vi "Unknown Signal State Machine.vi"() -> ()   [LabVIEW 2011]
doc: "Use this template to build a standard state machine design pattern. Each state executes code and determines which state to transition to. Contrast this design pattern with the User Interface Event Handler pattern, in which code executes in response to user actions. Contrast this design pattern also with the Queued Message Handler pattern, in which each message handling code can queue zero or more new messages."
uses:
  DAQstates.ctl
  <vilib>/DAQmx/read.llb/DAQmx Read (Analog 1D Wfm NChan NSamp).vi
  <vilib>/DAQmx/create/channels.llb/DAQmx Create Channel (AI-Voltage-Basic).vi
  <vilib>/DAQmx/configure/timing.llb/DAQmx Timing (Sample Clock).vi
  <vilib>/DAQmx/miscellaneous.llb/DAQmx Fill In Error Info.vi
  <vilib>/Waveform/WDTFileIO.llb/Export Waveforms To Spreadsheet File (1D).vi
panel:
  out "Waveform Graph":waveform(dbl)[](graph)
  out "Current State":T1
  in  "Stop":bool
  in  "Save Data":bool
  in  "Take Data":bool
  in  "Channel 2":tag
  in  "samples per channel":i32=1000
  in  "Rate(Hz)":dbl=1000.0 format="%0.2f"
  in  "Channel 1":tag
  out "Error Messages":errorcluster
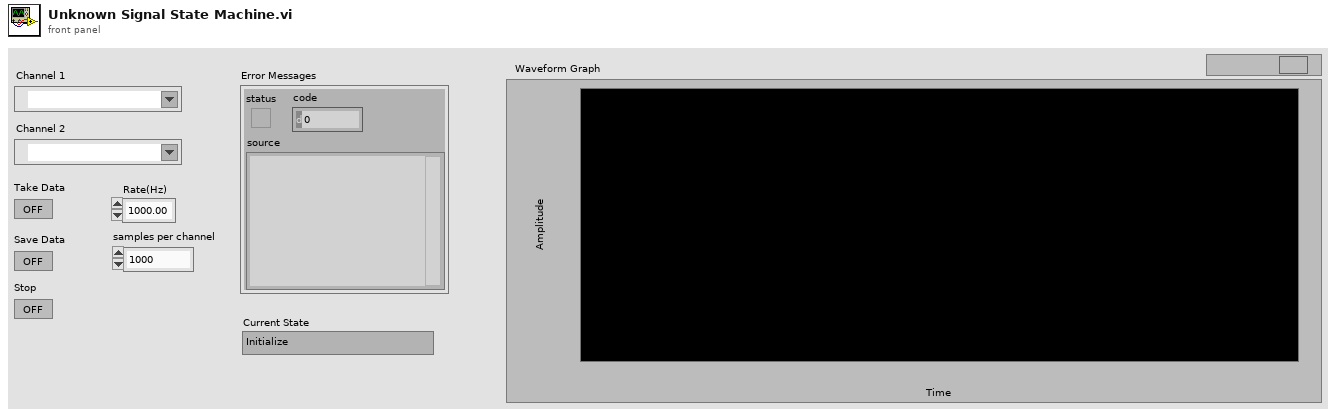
[diagram p1: front panel]
types:
  T1 = typedef "DAQstates.ctl" = enum16{"Initialize", "Wait", "Stop", "Take Data", "Save Data", ""}
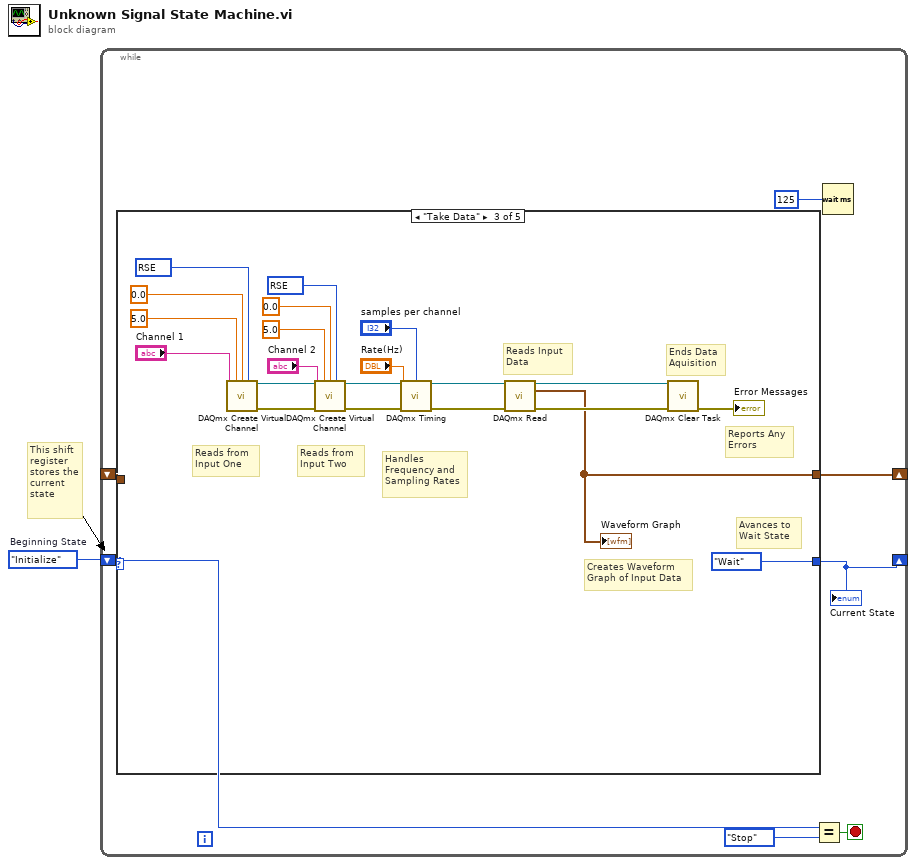
[diagram p0: block diagram]
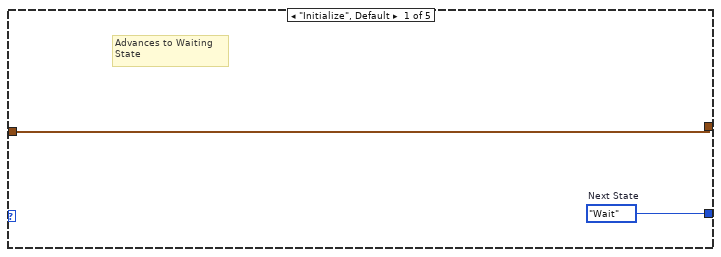
[diagram p2: hidden frame]
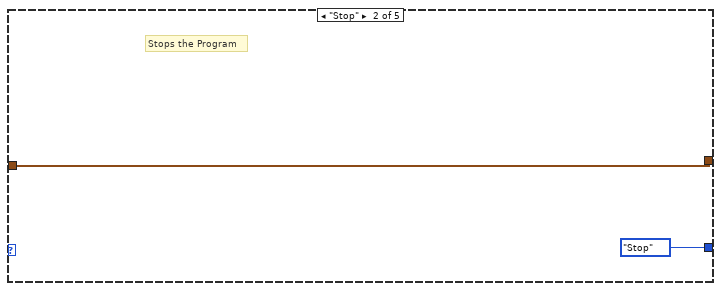
[diagram p3: hidden frame]
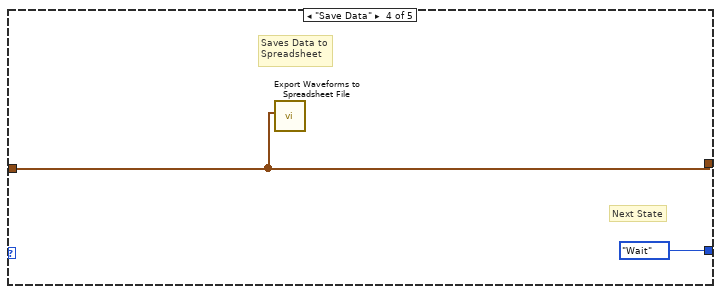
[diagram p4: hidden frame]
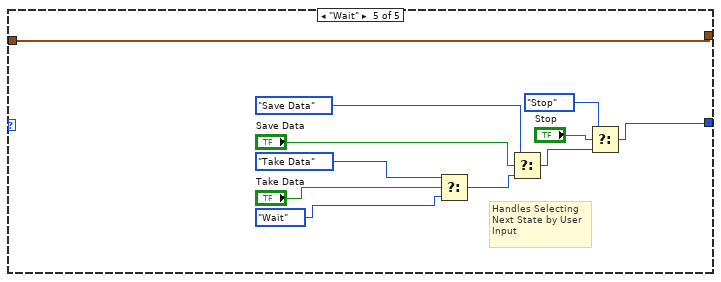
[diagram p5: hidden frame]
diagram:
  w1 = DAQstates."Initialize"  # Beginning State
  # "This shift\nregister\nstores the\ncurrent\nstate"
  n1 = while {
    shift-right: [w5] -> _
    shift-left: w1 -> [w6]
    shift-right: [w2] -> _
    shift-left: _ -> [w3]
    stop <- w8 stop-if-true
    n2 = case shown="\"Take Data\"" w6 {
      tunnel: [w10 DAQstates."Stop" ("Next State") DAQstates."Wait" ("Next State") DAQstates."Wait" ("Next State") w36] -> w5
      tunnel: [w9 w11 w14 w34 w46] -> w2
      tunnel: w3 -> [w9 w11 _ w34 w46]
      frame "Initialize", Default {
        w10 = DAQstates."Wait"  # Next State
        # "Advances to Waiting \nState"
      }
      frame "Stop" {
        # "Stops the Program"
      }
      frame "Take Data" {
        w23 = 10083 items=["default"=-1, "RSE"=10083, "NRSE"=10078, "Differential"=10106, "Pseudodifferential"=12529] ("input terminal configuration")
        w24 = 10083 items=["default"=-1, "RSE"=10083, "NRSE"=10078, "Differential"=10106, "Pseudodifferential"=12529] ("input terminal configuration")
        # "Reports Any\nErrors"
        # "Ends Data \nAquisition"
        # "Avances to \nWait State"
        # "Creates Waveform\nGraph of Input Data"
        # "Reads Input \nData"
        # "Handles\nFrequency and\nSampling Rates"
        # "Reads from \nInput Two"
        # "Reads from \nInput One"
        n3 = call-poly <vilib>:"DAQmx Create Virtual Channel.vi"("maximum value"=5.0, "minimum value"=0.0, "input terminal configuration"=w23, "physical channels"="Channel 1") -> ("task out"=w30:refnum<k21>, "error out"=w27:errorcluster)  [unwired: 10 in]
        n4 = call-poly <vilib>:"DAQmx Create Virtual Channel.vi"("task in"=w30, "maximum value"=5.0, "minimum value"=0.0, "input terminal configuration"=w24, "physical channels"="Channel 2", "error in"=w27) -> ("task out"=w20:refnum<k21>, "error out"=w19:errorcluster)  [unwired: 8 in]
        n5 = call-poly <vilib>:"DAQmx Timing.vi"("task/channels in"=w20, "samples per channel"="samples per channel", "rate"="Rate(Hz)", "error in"=w19) -> ("task out"=w17:refnum<k21>, "error out"=w18:errorcluster)  [unwired: 10 in]
        n6 = call-poly <vilib>:"DAQmx Read.vi"("task/channels in"=w17, "error in"=w18) -> ("task out"=w16:refnum<k21>, "data"=w14:waveform(dbl)[], "error out"=w15:errorcluster)  [unwired: 11 in]
        "Waveform Graph" <- w14
        n7 = call <vilib>:"DAQmx Clear Task.vi"("task in"=w16, "error in"=w15) -> ("error out"=→"Error Messages":errorcluster)  [unwired: 13 in]
      }
      frame "Save Data" {
        # "Next State"
        # "Saves Data to\nSpreadsheet"
        n8 = call-poly <vilib>:"Export Waveforms to Spreadsheet File.vi"("waveforms"=w34) -> ()  [unwired: 9 in, 2 out]
      }
      frame "Wait" {
        # "Handles Selecting\nNext State by User \nInput"
        n9 = Select(t=DAQstates."Take Data" ("Next State"), s="Take Data", f=DAQstates."Wait" ("Next State")) -> (s? t:f=w42:T1)
        n10 = Select(t=DAQstates."Save Data" ("Next State"), s="Save Data", f=w42) -> (s? t:f=w39:T1)
        n11 = Select(t=DAQstates."Stop", s="Stop", f=w39) -> (s? t:f=w36:T1)
      }
    }
    "Current State" <- w5
    n12 = Equal?(x=w6, y=DAQstates."Stop" ("States")) -> (x = y?=w8:bool)
    n13 = Wait (ms)(milliseconds to wait=u32 125) -> ()  [unwired: 1 out]
  }
